vi "Get Seed Locations.vi"(1 "Maps":T1(c390), 2 "Seeds":u64[](array[numeric])) -> (0 "Locations":u64[](array[numeric]))   [LabVIEW 2020, in "AoC 2023.lvlib"]
uses:
  AoC 2023.lvlib
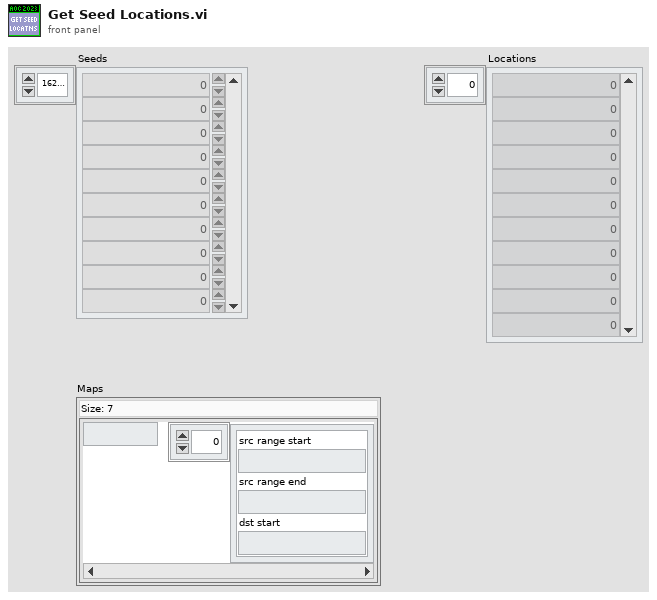
[diagram p1: front panel]
types:
  T1 = map{i32, cluster{"src range start":u64, "src range end":u64, "dst start":u64}[]}
  T2 = cluster{"src range start":u64, "src range end":u64, "dst start":u64}[]
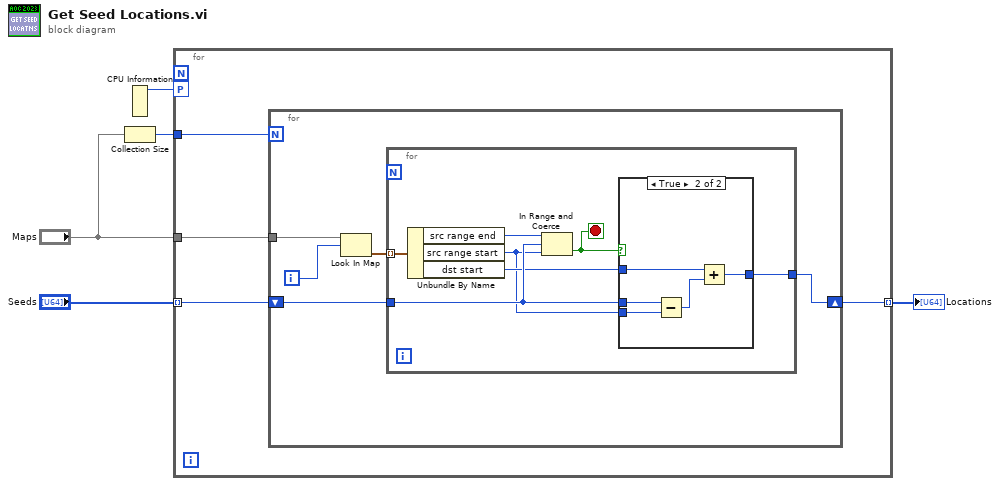
[diagram p0: block diagram]
diagram:
  n1 = CPU Information() -> (4:w1:i32)  [unwired: 3 out]
  n2 = Collection Size(1:"Maps") -> (0:w4:i32)
  n3 = for {
    tunnel: "Seeds" -> [w7] mode=indexing
    tunnel: "Maps" -> [w9]
    tunnel: w4 -> [w8]
    tunnel: [w6] -> w5 mode=indexing
    workers-P: w1 -> [_]
    n4 = for {
      N: w8 -> [_]
      tunnel: w9 -> [w10]
      shift-right: [w12] -> w6
      shift-left: w7 -> [w13]
      i -> [w14]
      n5 = Look In Map(map=w10, key=w14) -> (value=w11:T2)  [unwired: 1 in, 1 out]
      n6 = for {
        tunnel: w11 -> [w21] mode=indexing
        tunnel: w13 -> [w20]
        tunnel: [w17] -> w12
        stop <- w16 stop-if-true
        n7 = Unbundle By Name(w21) -> ("src range end"=w19:u64, "src range start"=w15:u64, "dst start"=w18:u64)
        n8 = In Range and Coerce(upper limit=w19, x=w20, lower limit=w15) -> (In Range?=w16:bool)  [unwired: 1 out]
        n9 = case shown="True" w16 {
          tunnel: w20 -> [w22 w27]
          tunnel: w15 -> [_ w26]
          tunnel: w18 -> [_ w25]
          tunnel: [w22 w23] -> w17
          frame False {
          }
          frame True {
            n10 = Subtract(x=w27, y=w26) -> (x-y=w24:u64)
            n11 = Add(x=w25, y=w24) -> (x+y=w23:u64)
          }
        }
      }
    }
  }
  "Locations" <- w5
